vi "BroadcastPositionData.vi"(3 "error in (no error)":errorcluster, 4 "Simulated Satellite Data":T1={"Position Array"=[[10, 100], [500, 1000], [90, 270]], "Target Names"=["R", "G", "B", "Q", "R", "S", "T"]}, 5 "connection ID":refnum<k16>) -> (0 "error out":errorcluster, 1 "Data sent":string, 2 "connection ID out":refnum<k16>)   [LabVIEW 2012]
panel:
  out "Example Data Sent (data rec'd)":string="$,G,274,67,B,245,67,R,255,42,N,282,44,S,14,5,395\r"
  # "SIMULATED BASE STATION"
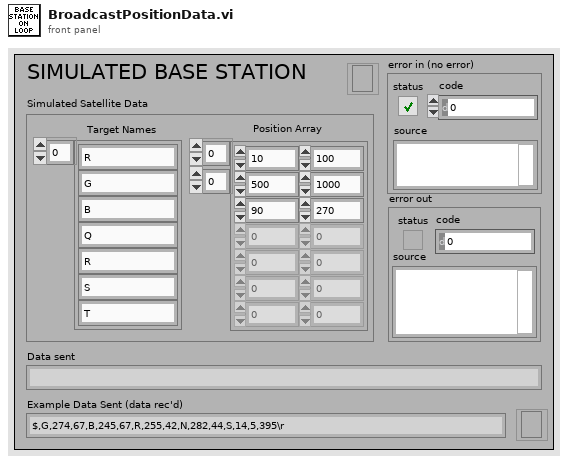
[diagram p1: front panel]
types:
  T1 = cluster{"Position Array":i32[][], "Target Names":string[]}
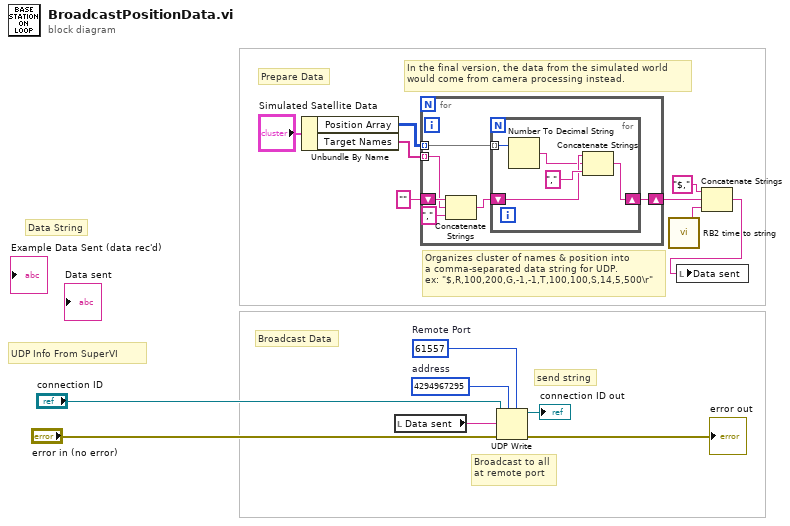
[diagram p0: block diagram]
diagram:
  w6 = u16 61557  # Remote Port
  w5 = u32 4294967295  # address
  # "Data String"
  # "Broadcast Data"
  # "send string"
  # "Broadcast to all\nat remote port"
  # "UDP Info From SuperVI"
  # "Organizes cluster of names & position into\na comma-separated data string for UDP.\nex: \"$,R,100,200,G,-1,-1,T,100,100,S,14,5,500\\r\""
  # "In the final version, the data from the simulated world\nwould come from camera processing instead."
  # "Prepare Data"
  n1 = Unbundle By Name("Simulated Satellite Data") -> ("Position Array"=w12:i32[][], "Target Names"=w11:string[])
  n2 = local read "Data sent"() -> (w4:string)
  n3 = for {
    shift-right: [w20] -> w9
    shift-left: "" -> [w18]
    tunnel: w12 -> [w21] mode=indexing
    tunnel: w11 -> [w17] mode=indexing
    n4 = Concatenate Strings(w18, w17, "," ("string")) -> (w16:string)
    n5 = for {
      shift-right: [w24] -> w20
      shift-left: w16 -> [w25]
      tunnel: w21 -> [w23] mode=indexing
      n6 = Number To Decimal String(number=w23) -> (decimal integer string=w22:string)  [unwired: 1 in]
      n7 = Concatenate Strings(w25, w22, "," ("string")) -> (w24:string)
    }
  }
  n8 = UDP Write(address=w5, port or service name=w6, connection ID="connection ID", data in=w4, 8:"error in (no error)") -> (error out=→"error out":errorcluster, 3:→"connection ID out":refnum<k16>)  [unwired: 1 out]
  n9 = call "RB2 time to string.vi"() -> ("time string"=w7:string)  [unwired: 1 in]
  n10 = Concatenate Strings("$," ("string"), w9, w7) -> (w10:string)
  n11 = local write "Data sent"(w10) -> ()
